vi "Test.vi"() -> ()   [LabVIEW 2012]
uses:
  Opening Purpose.ctl
panel:
  out "error out":errorcluster
  in  "Original File Path":path
  in  "Opening Purpose":T1
  in  "TIFF File Path":path
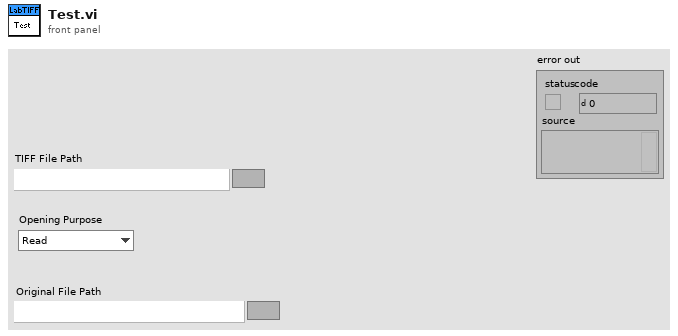
[diagram p1: front panel]
types:
  T1 = typedef "Opening Purpose.ctl" = enum16{"Read", "Write"}
  T2 = typedef "Image Type" = u32
  T3 = typedef "IMAQ Image.ctl" = refnum<image>
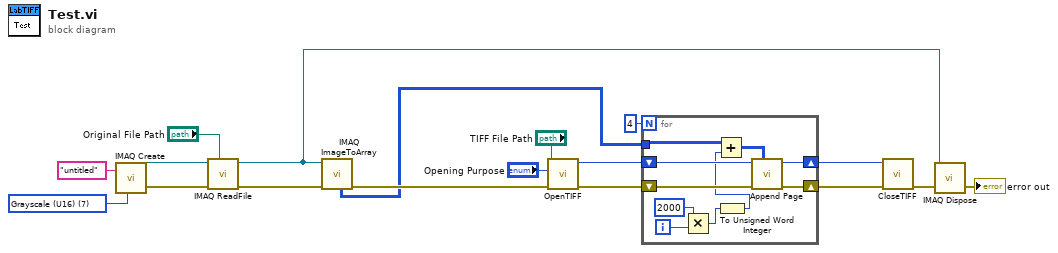
[diagram p0: block diagram]
diagram:
  w13 = T2 7 items=["Grayscale (U8)", "Grayscale (I16)", "Grayscale (SGL)", "Complex (CSG)", "RGB (U32)", "HSL (U32)", "RGB (U64)", "Grayscale (U16)"] ("Image Type")
  n1 = call "IMAQ Create"("Image Name"="untitled", "Image Type"=w13) -> ("New Image"=w15:T3, "error out"=w14:errorcluster)  [unwired: 3 in]
  n2 = call "IMAQ ReadFile"("File Path"="Original File Path", "error in (no error)"=w14, "Image"=w15) -> ("error out"=w11:errorcluster, "Image Out"=w4:T3)  [unwired: 4 in, 3 out]
  n3 = call "IMAQ ImageToArray"("error in (no error)"=w11, "Image"=w4) -> ("Image Pixels (U16)"=w2:u16[][], "error out"=w10:errorcluster)  [unwired: 2 in, 3 out]
  n4 = call "OpenTIFF.vi"("error in (no error)"=w10, "Opening Purpose"="Opening Purpose", "File Path"="TIFF File Path") -> ("error out"=w9:errorcluster, "TIFF File Ref"=w8:i32)  [unwired: 7 in]
  n5 = for {
    N: 4 -> [_]
    tunnel: w2 -> [w22]
    shift-right: [w26] -> w6
    shift-left: w9 -> [w28]
    shift-right: [w27] -> w7
    shift-left: w8 -> [w23]
    i -> [w25]
    n6 = Multiply(x=2000, y=w25) -> (x*y=w21:i32)
    n7 = To Unsigned Word Integer(number=w21) -> (unsigned 16bit integer=w20:u16)
    n8 = Add(x=w22, y=w20) -> (x+y=w19:u16[][])
    n9 = call "Append Page.vi"("U16 Image"=w19, "error in (no error)"=w28, "TIFF File Ref"=w23) -> ("error out"=w26:errorcluster, "TIFF File Ref out"=w27:i32)  [unwired: 7 in]
  }
  n10 = call "CloseTIFF.vi"("error in (no error)"=w6, "TIFF File Ref"=w7) -> ("error out"=w5:errorcluster)  [unwired: 9 in]
  n11 = call "IMAQ Dispose"("Image"=w4, "error in (no error)"=w5) -> ("error out"=→"error out":errorcluster)  [unwired: 4 in]
